vi "Read SHH Coeffs.vi"(8 "error in (no error)":errorcluster, 11 "Open Path CRD in":refnum<class "Open Path CRD.lvclass">) -> (0 "error out":errorcluster, 2 "SHH Coeffs":dbl[][](array[numeric]), 3 "Open Path CRD out":refnum<class "Open Path CRD.lvclass">)   [LabVIEW 2015, in "Open Path CRD.lvclass"]
uses:
  Open Path CRD.lvclass
  Open Path CRD.lvclass/Open Path CRD.ctl
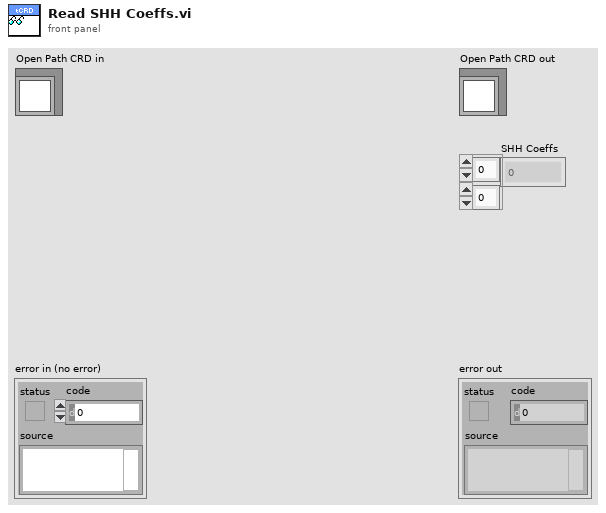
[diagram p1: front panel]
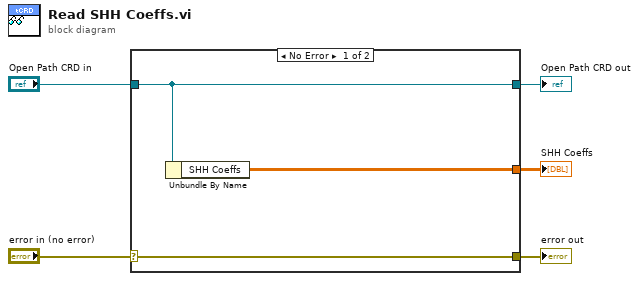
[diagram p0: block diagram]
diagram:
  n1 = case shown="No Error" "error in (no error)" {
    selector: "error in (no error)" -> [w8 w9]
    tunnel: [w8 w9] -> w4
    tunnel: [w7 w10] -> w2
    tunnel: "Open Path CRD in" -> [w7 w10]
    tunnel: [w6 _] -> w1
    frame No Error {
      n2 = Unbundle By Name(w7) -> ("SHH Coeffs"=w6:dbl[][])
    }
    frame Error {
    }
  }
  "error out" <- w4
  "Open Path CRD out" <- w2
  "SHH Coeffs" <- w1
